vi "Set Protocol Data.vi"(7 "Operation":T1, 8 "error in (no error)":errorcluster, 10 "Protocols.lvlib:Protocol Parent.lvclass":refnum<class "Protocol Parent.lvclass">, 11 "Listener In.lvclass":refnum<class "Listener.lvclass"> caption="Listener") -> (0 "error out":errorcluster, 3 "Listener Out.lvclass":refnum<class "Listener.lvclass">)   [LabVIEW 2023, in "Listener.lvclass"]
uses:
  Listener.lvclass
  TCP/TCP.lvclass
  UDP/UDP.lvclass
  ListenerClassControls/TCP Data Structure.ctl
  ListenerClassControls/UDP Data Structure.ctl
  AK TCP/AK TCP.lvclass
  ListenerClassControls/AK TCP Data Structure.ctl
  ListenerClassControls/Protocol.ctl
  Constants.vi
  AK RS-xxx/AK RS-xxx.lvclass
  ListenerClassControls/RS-xxx Data Structure.ctl
  Protocol Parent/Protocol Parent.lvclass
  <vilib>/Instr/_visa.llb/VISA Configure Serial Port (Instr).vi
  ListenerClassControls/Operation.ctl
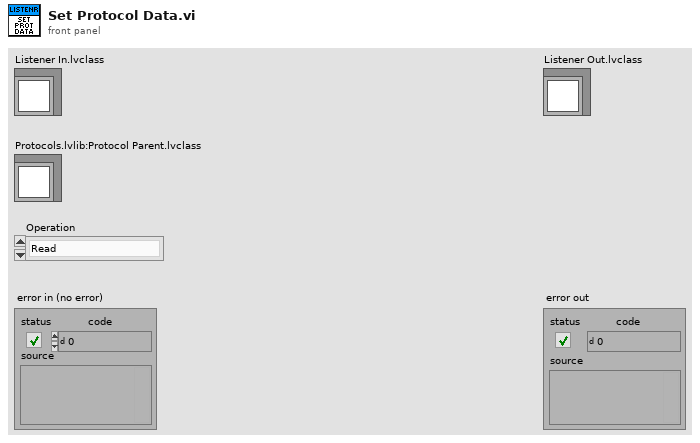
[diagram p1: front panel]
types:
  T1 = typedef "Listener.lvclass/Operation.ctl" = enum16{"Read", "Write"}
  T2 = typedef "Listener.lvclass/Protocol.ctl" = enum16{"RS-XXX", "AK RS-XXX", "VISA", "TCPIP", "AK TCPIP", "UDP", "GPIB ConvBox"}
  T3 = typedef "Listener.lvclass/AK TCP Data Structure.ctl" = cluster{"TCP|IP connection ID":refnum<k5>, "IP Address":string, "Port":u16, "Data":string, "Current Command Code":string}
  T4 = typedef "Listener.lvclass/TCP Data Structure.ctl" = cluster{"TCP|IP connection ID":refnum<k5>, "IP Address":string, "Port":u16, "Data":string}
  T5 = typedef "Listener.lvclass/UDP Data Structure.ctl" = cluster{"UDP connection ID":refnum<k16>, "Local Address":string, "Local Port":u16, "Target IP Address":string, "Target Port":u16, "Data":string}
  T6 = typedef "Listener.lvclass/RS-xxx Data Structure.ctl" = cluster{"Virtual COM Port Settings 1":cluster{"Port":string, "Baud Rate":u32, "Data Bits":u16, "Parity":enum16{"None", "Odd", "Even", "Mark", "Space"}, "Stop Bits":u16, "Flow Control":u16, "XON":enum16{"NUL", "SOH", "STX", "ETX", "EOT", "ENQ", "ACK", "BEL", "BS", "HT", "LF", "VT", "FF", "CR", "SO", "SI", "DLE", "DC1", "DC2", "DC3", "DC4", "NAK", "SYN", "ETB", "CAN", "EM", "SUB", "ESC", "FS", "GS", "RS", "US", "SP", "!", "\"", "#", "$", "%", "&", "'", "(", ")", "*", "+", ",", "- (-)", ".", "/", "0", "1", "2", "3", "4", "5", "6", "7", "8", "9", ":", ";", "<", "=", ">", "?", "@", "A", "B", "C", "D", "E", "F", "G", "H", "I", "J", "K", "L", "M", "N", "O", "P", "Q", "R", "S", "T", "U", "V", "W", "X", "Y", "Z", "[", "\\", "]", "^", "_", "`", "a", "b", "c", "d", "e", "f", "g", "h", "i", "j", "k", "l", "m", "n", "o", "p", "q", "r", "s", "t", "u", "v", "w", "x", "y", "z", "{", "|", "}", "~"}, "XOFF":enum16{"NUL", "SOH", "STX", "ETX", "EOT", "ENQ", "ACK", "BEL", "BS", "HT", "LF", "VT", "FF", "CR", "SO", "SI", "DLE", "DC1", "DC2", "DC3", "DC4", "NAK", "SYN", "ETB", "CAN", "EM", "SUB", "ESC", "FS", "GS", "RS", "US", "SP", "!", "\"", "#", "$", "%", "&", "'", "(", ")", "*", "+", ",", "- (-)", ".", "/", "0", "1", "2", "3", "4", "5", "6", "7", "8", "9", ":", ";", "<", "=", ">", "?", "@", "A", "B", "C", "D", "E", "F", "G", "H", "I", "J", "K", "L", "M", "N", "O", "P", "Q", "R", "S", "T", "U", "V", "W", "X", "Y", "Z", "[", "\\", "]", "^", "_", "`", "a", "b", "c", "d", "e", "f", "g", "h", "i", "j", "k", "l", "m", "n", "o", "p", "q", "r", "s", "t", "u", "v", "w", "x", "y", "z", "{", "|", "}", "~"}, "End Read on Termination Character":bool, "End Write on Termination Character":bool, "Termination Character":u8}, "Virtual COM Port Settings 2":cluster{"Port":string, "Baud Rate":u32, "Data Bits":u16, "Parity":enum16{"None", "Odd", "Even", "Mark", "Space"}, "Stop Bits":u16, "Flow Control":u16, "XON":enum16{"NUL", "SOH", "STX", "ETX", "EOT", "ENQ", "ACK", "BEL", "BS", "HT", "LF", "VT", "FF", "CR", "SO", "SI", "DLE", "DC1", "DC2", "DC3", "DC4", "NAK", "SYN", "ETB", "CAN", "EM", "SUB", "ESC", "FS", "GS", "RS", "US", "SP", "!", "\"", "#", "$", "%", "&", "'", "(", ")", "*", "+", ",", "- (-)", ".", "/", "0", "1", "2", "3", "4", "5", "6", "7", "8", "9", ":", ";", "<", "=", ">", "?", "@", "A", "B", "C", "D", "E", "F", "G", "H", "I", "J", "K", "L", "M", "N", "O", "P", "Q", "R", "S", "T", "U", "V", "W", "X", "Y", "Z", "[", "\\", "]", "^", "_", "`", "a", "b", "c", "d", "e", "f", "g", "h", "i", "j", "k", "l", "m", "n", "o", "p", "q", "r", "s", "t", "u", "v", "w", "x", "y", "z", "{", "|", "}", "~"}, "XOFF":enum16{"NUL", "SOH", "STX", "ETX", "EOT", "ENQ", "ACK", "BEL", "BS", "HT", "LF", "VT", "FF", "CR", "SO", "SI", "DLE", "DC1", "DC2", "DC3", "DC4", "NAK", "SYN", "ETB", "CAN", "EM", "SUB", "ESC", "FS", "GS", "RS", "US", "SP", "!", "\"", "#", "$", "%", "&", "'", "(", ")", "*", "+", ",", "- (-)", ".", "/", "0", "1", "2", "3", "4", "5", "6", "7", "8", "9", ":", ";", "<", "=", ">", "?", "@", "A", "B", "C", "D", "E", "F", "G", "H", "I", "J", "K", "L", "M", "N", "O", "P", "Q", "R", "S", "T", "U", "V", "W", "X", "Y", "Z", "[", "\\", "]", "^", "_", "`", "a", "b", "c", "d", "e", "f", "g", "h", "i", "j", "k", "l", "m", "n", "o", "p", "q", "r", "s", "t", "u", "v", "w", "x", "y", "z", "{", "|", "}", "~"}, "End Read on Termination Character":bool, "End Write on Termination Character":bool, "Termination Character":u8}, "Data":string, "Data Length":u32}
  T7 = typedef "Protocols.lvlib/Protocol Parent.lvclass/Base Protocol Type.ctl" = enum16{"RS-XXX", "VISA", "TCPIP", "UDP", "GPIB ConvBox"}
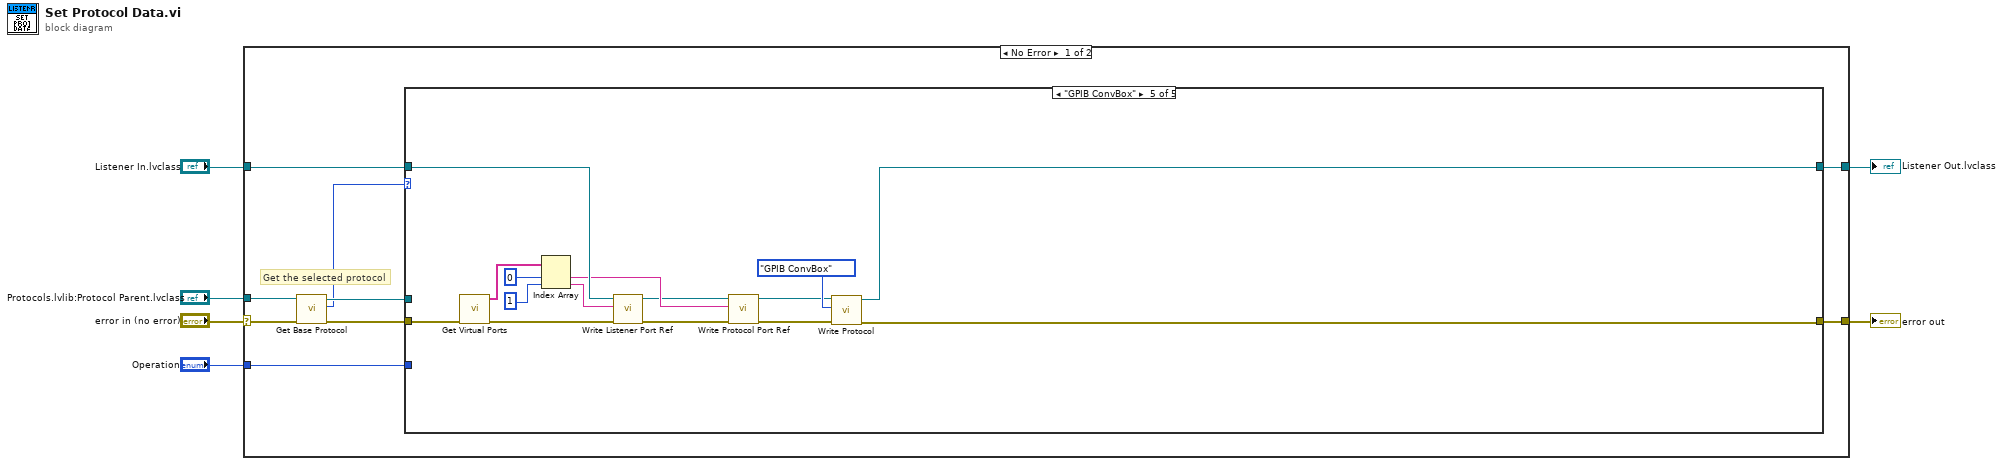
[diagram p0: block diagram]
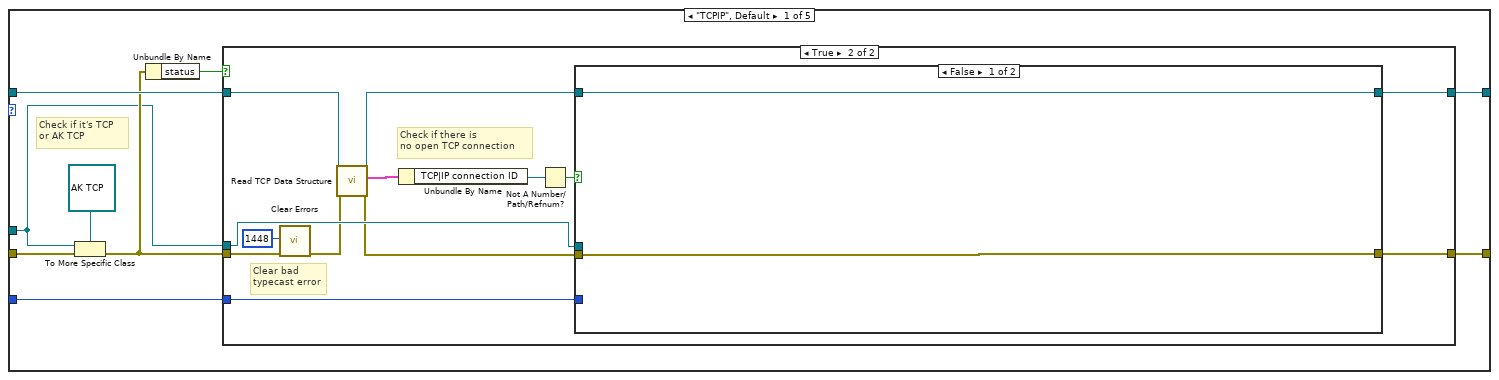
[diagram p2: hidden frame]
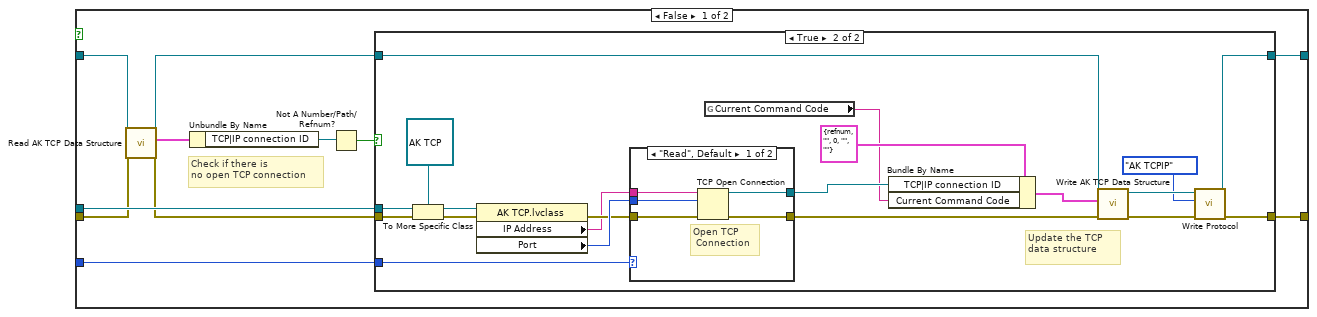
[diagram p3: hidden frame]
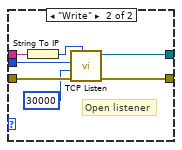
[diagram p5: hidden frame]
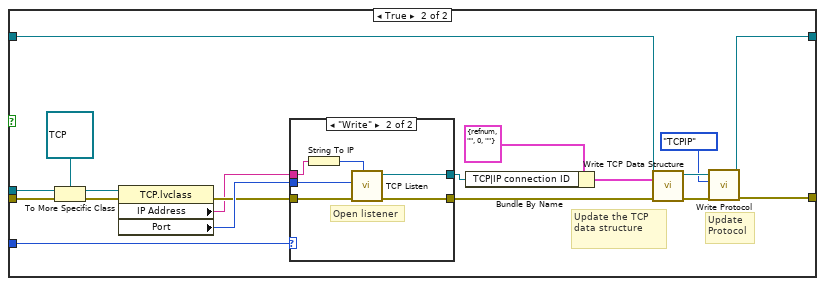
[diagram p6: hidden frame]
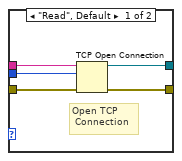
[diagram p7: hidden frame]
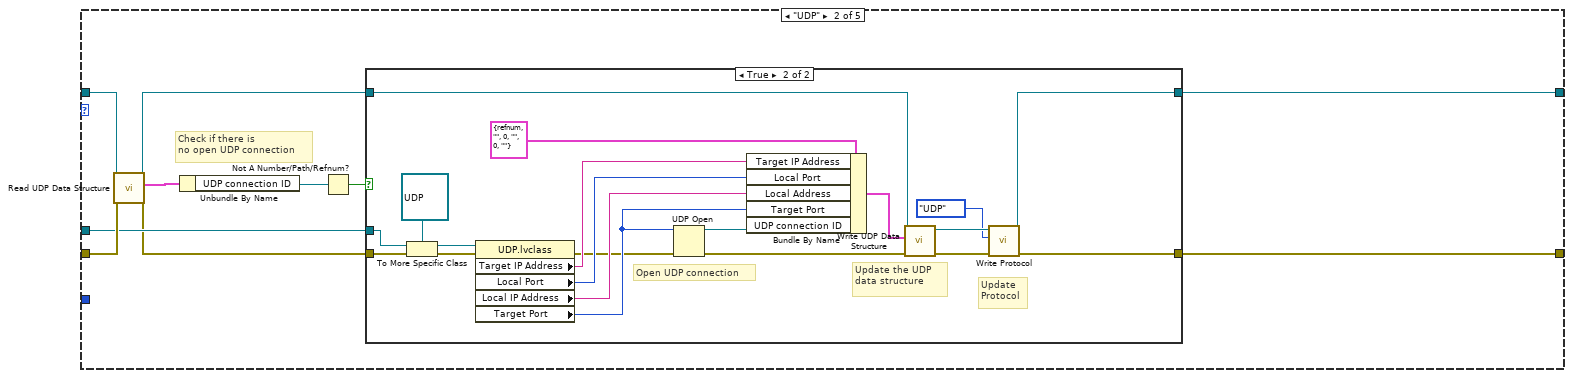
[diagram p8: hidden frame]
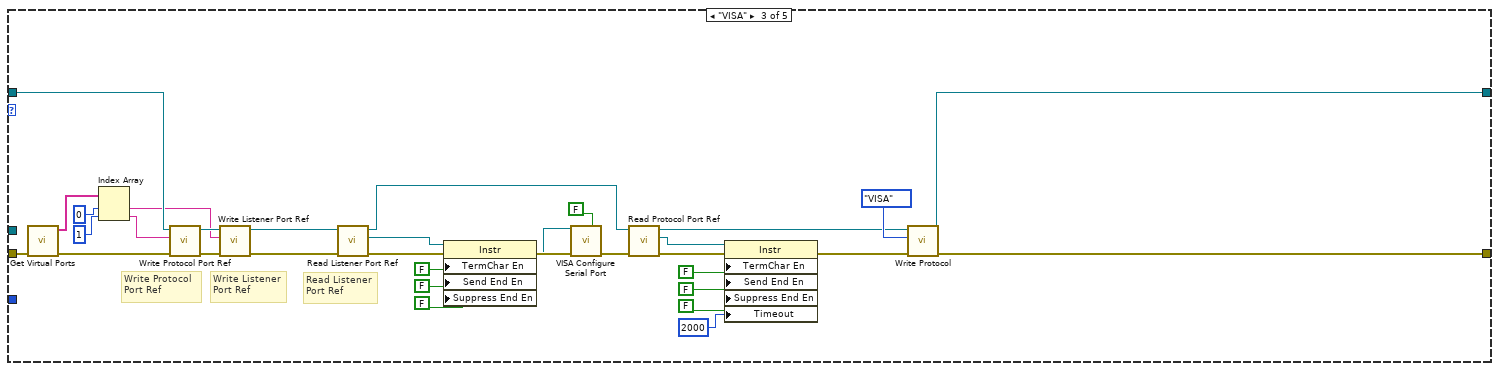
[diagram p10: hidden frame]
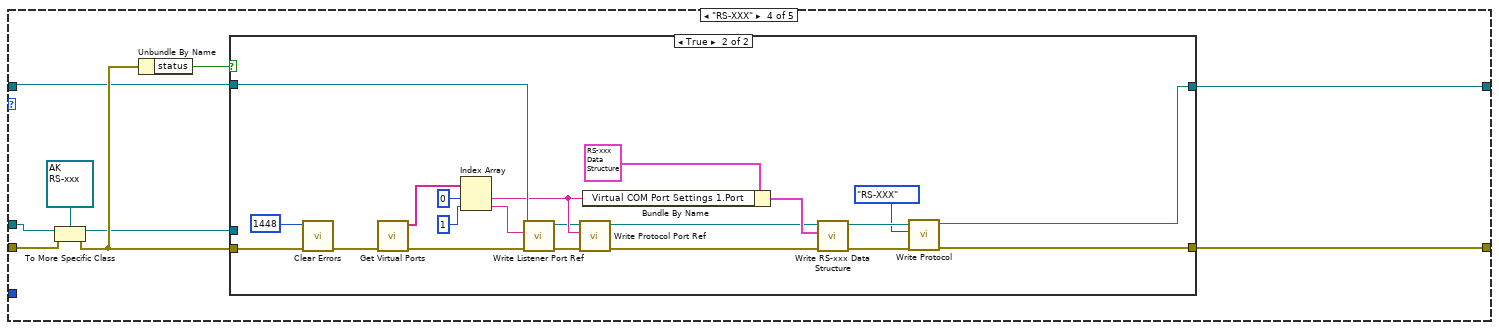
[diagram p11: hidden frame]
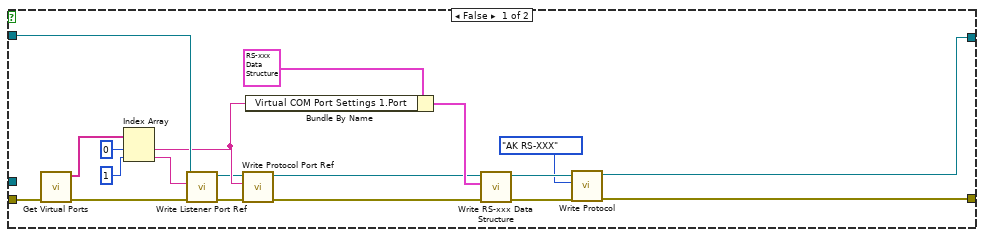
[diagram p12: hidden frame]
diagram:
  n1 = case shown="No Error" "error in (no error)" {
    selector: "error in (no error)" -> [w13 w245]
    tunnel: [w12 w245] -> w5
    tunnel: "Protocols.lvlib:Protocol Parent.lvclass" -> [w14 _]
    tunnel: "Listener In.lvclass" -> [w7 w244]
    tunnel: [w9 w244] -> w2
    tunnel: "Operation" -> [w8 _]
    frame No Error {
      # "Get the selected protocol"
      n2 = call-dynamic "Get Base Protocol.vi"("error in (no error)"=w13, "Protocol Parent in"=w14) -> ("error out"=w11:errorcluster, "Protocol out"=w10:T7, "Protocol Parent out"=w15:refnum<class "Protocol Parent.lvclass">)  [unwired: 7 in]
      n3 = case shown="\"GPIB ConvBox\"" w10 {
        tunnel: w15 -> [w16 w118 _ w181 _]
        tunnel: w11 -> [w20 w120 w179 w188 w243]
        tunnel: [w23 w123 w165 w183 w242] -> w12
        tunnel: w7 -> [w22 w119 w154 w184 w236]
        tunnel: [w24 w124 w178 w182 w241] -> w9
        tunnel: w8 -> [w21 _ _ _ _]
        frame "TCPIP", Default {
          # "Check if it's TCP \nor AK TCP"
          n4 = To More Specific Class(target class=refnum<class "AK TCP.lvclass"> refnum ("Protocols.lvlib:AK TCP.lvclass"), reference=w16, error in=w20) -> (error out=w19:errorcluster)  [unwired: 1 out]
          n5 = Unbundle By Name(w19) -> ("status"=w18:bool)
          n6 = case shown="True" w18 {
            tunnel: w16 -> [w35 w82]
            tunnel: [w34 w81] -> w24
            tunnel: [w33 w80] -> w23
            tunnel: w22 -> [w30 w78]
            tunnel: w19 -> [w28 w77]
            tunnel: w21 -> [w31 w72]
            frame False {
              # "Check if there is \nno open TCP connection"
              n7 = call-dynamic "Read AK TCP Data Structure.vi"("error in (no error)"=w28, "Listener in"=w30) -> ("error out"=w27:errorcluster, "TCP|IP Data Structure"=w26:T3, "Listener out"=w29:refnum<class "Listener.lvclass">)  [unwired: 7 in]
              n8 = Unbundle By Name(w26) -> ("TCP|IP connection ID"=w25:refnum<k5>)
              n9 = Not A Number/Path/Refnum?(number/path/refnum=w25) -> (NaN/Path/Refnum?=w32:bool)
              n10 = case shown="True" w32 {
                tunnel: w35 -> [_ w57]
                tunnel: [w37 w38] -> w34
                tunnel: [w36 w41] -> w33
                tunnel: w27 -> [w36 w54]
                tunnel: w29 -> [w37 w43]
                tunnel: w31 -> [_ w53]
                frame False {
                }
                frame True {
                  # "Update the TCP \ndata structure"
                  n11 = To More Specific Class(target class=refnum<class "AK TCP.lvclass"> refnum ("Protocols.lvlib:AK TCP.lvclass"), reference=w57, error in=w54) -> (specific class reference=w56:refnum<class "AK TCP.lvclass">, error out=w55:errorcluster)
                  n12 = property class="AK TCP.lvclass"(reference=w56, error in=w55) -> (error out=w51:errorcluster, "IP Address"=w50:string, "Port"=w52:u16)  [unwired: 1 out]
                  n13 = case shown="\"Read\", Default" w53 {
                    tunnel: w52 -> [w62 w64]
                    tunnel: w51 -> [w61 w69]
                    tunnel: w50 -> [w60 w68]
                    tunnel: [w59 w65] -> w45
                    tunnel: [w58 w66] -> w49
                    frame "Read", Default {
                      # "Open TCP\n Connection"
                      n14 = TCP Open Connection(address=w60, remote port or service name=w62, error in (no error)=w61) -> (connection ID=w58:refnum<k5>, error out=w59:errorcluster)  [unwired: 2 in]
                    }
                    frame "Write" {
                      # "Open listener"
                      n15 = String To IP(1:w68) -> (0:w67:u32)
                      n16 = call <vilib>:"TCP Listen.vi"("net address"=w67, "error in (no error)"=w69, "timeout ms (wait forever: -1)"=30000, "port"=w64) -> ("error out"=w65:errorcluster, "connection ID"=w66:refnum<k5>)  [unwired: 3 in, 3 out]
                    }
                  }
                  n17 = global read "Constants.vi" "Current Command Code"() -> (w46:string)
                  n18 = Bundle By Name(cluster=T3 {"TCP|IP connection ID"=refnum, "IP Address"="", "Port"=0, "Data"="", "Current Command Code"=""} ("TCP|IP Data Structure"), "TCP|IP connection ID"=w49, "Current Command Code"=w46) -> (w44:T3)
                  n19 = call-dynamic "Write AK TCP Data Structure.vi"("error in (no error)"=w45, "TCP|IP Data Structure"=w44, "Listener in"=w43) -> ("error out"=w42:errorcluster, "Listener out"=w40:refnum<class "Listener.lvclass">)  [unwired: 7 in]
                  n20 = call-dynamic "Write Protocol.vi"("error in (no error)"=w42, "Protocol"=Protocol."AK TCPIP", "Listener in"=w40) -> ("error out"=w41:errorcluster, "Listener out"=w38:refnum<class "Listener.lvclass">)  [unwired: 7 in]
                }
              }
            }
            frame True {
              # "Clear bad \ntypecast error"
              # "Check if there is \nno open TCP connection"
              n21 = call <vilib>:"Clear Errors.vi"("error in (no error)"=w77, "specific error code to clear (0: all)"=1448) -> ("error out"=w71:errorcluster)  [unwired: 4 in, 1 out]
              n22 = call-dynamic "Read TCP Data Structure.vi"("error in (no error)"=w71, "Listener in"=w78) -> ("error out"=w76:errorcluster, "TCP|IP Data Structure"=w75:T4, "Listener out"=w74:refnum<class "Listener.lvclass">)  [unwired: 7 in]
              n23 = Unbundle By Name(w75) -> ("TCP|IP connection ID"=w79:refnum<k5>)
              n24 = Not A Number/Path/Refnum?(number/path/refnum=w79) -> (NaN/Path/Refnum?=w73:bool)
              n25 = case shown="False" w73 {
                tunnel: w82 -> [_ w102]
                tunnel: [w84 w86] -> w81
                tunnel: [w83 w87] -> w80
                tunnel: w76 -> [w83 w98]
                tunnel: w74 -> [w84 w91]
                tunnel: w72 -> [_ w97]
                frame False {
                }
                frame True {
                  # "Update \nProtocol"
                  # "Update the TCP \ndata structure"
                  n26 = To More Specific Class(target class=refnum<class "TCP.lvclass"> refnum ("Protocols.lvlib:TCP.lvclass"), reference=w102, error in=w98) -> (specific class reference=w101:refnum<class "TCP.lvclass">, error out=w100:errorcluster)
                  n27 = property class="TCP.lvclass"(reference=w101, error in=w100) -> (error out=w95:errorcluster, "IP Address"=w94:string, "Port"=w96:u16)  [unwired: 1 out]
                  n28 = case shown="\"Write\"" w97 {
                    tunnel: w96 -> [w108 w113]
                    tunnel: w95 -> [w107 w114]
                    tunnel: w94 -> [w106 w112]
                    tunnel: [w105 w109] -> w92
                    tunnel: [w104 w110] -> w93
                    frame "Read", Default {
                      # "Open TCP\n Connection"
                      n29 = TCP Open Connection(address=w106, remote port or service name=w108, error in (no error)=w107) -> (connection ID=w104:refnum<k5>, error out=w105:errorcluster)  [unwired: 2 in]
                    }
                    frame "Write" {
                      # "Open listener"
                      n30 = String To IP(1:w112) -> (0:w111:u32)
                      n31 = call <vilib>:"TCP Listen.vi"("net address"=w111, "error in (no error)"=w114, "port"=w113) -> ("error out"=w109:errorcluster, "connection ID"=w110:refnum<k5>)  [unwired: 4 in, 3 out]
                    }
                  }
                  n32 = Bundle By Name(cluster=T4 {"TCP|IP connection ID"=refnum, "IP Address"="", "Port"=0, "Data"=""} ("TCP|IP Data Structure"), "TCP|IP connection ID"=w93) -> (w90:T4)
                  n33 = call-dynamic "Write TCP Data Structure.vi"("error in (no error)"=w92, "TCP|IP Data Structure"=w90, "Listener in"=w91) -> ("error out"=w89:errorcluster, "Listener out"=w88:refnum<class "Listener.lvclass">)  [unwired: 7 in]
                  n34 = call-dynamic "Write Protocol.vi"("error in (no error)"=w89, "Protocol"=Protocol."TCPIP", "Listener in"=w88) -> ("error out"=w87:errorcluster, "Listener out"=w86:refnum<class "Listener.lvclass">)  [unwired: 7 in]
                }
              }
            }
          }
        }
        frame "UDP" {
          # "Check if there is \nno open UDP connection"
          n35 = call-dynamic "Read UDP Data Structure.vi"("error in (no error)"=w120, "Listener in"=w119) -> ("error out"=w116:errorcluster, "UDP Data Structure"=w117:T5, "Listener out"=w115:refnum<class "Listener.lvclass">)  [unwired: 7 in]
          n36 = Unbundle By Name(w117) -> ("UDP connection ID"=w121:refnum<k16>)
          n37 = Not A Number/Path/Refnum?(number/path/refnum=w121) -> (NaN/Path/Refnum?=w122:bool)
          n38 = case shown="True" w122 {
            tunnel: w116 -> [w126 w146]
            tunnel: w118 -> [_ w144]
            tunnel: w115 -> [w125 w133]
            tunnel: [w125 w127] -> w124
            tunnel: [w126 w128] -> w123
            frame False {
            }
            frame True {
              # "Update \nProtocol"
              # "Update the UDP \ndata structure"
              # "Open UDP connection"
              n39 = To More Specific Class(target class=refnum<class "UDP.lvclass"> refnum ("Protocols.lvlib:UDP.lvclass"), reference=w144, error in=w146) -> (specific class reference=w138:refnum<class "UDP.lvclass">, error out=w143:errorcluster)
              n40 = property class="UDP.lvclass"(reference=w138, error in=w143) -> (error out=w136:errorcluster, "Target IP Address"=w142:string, "Local Port"=w141:u16, "Local IP Address"=w140:string, "Target Port"=w137:u16)  [unwired: 1 out]
              n41 = UDP Open(8:w136, 11:w137) -> (port=w135:refnum<k16>, 0:w134:errorcluster)  [unwired: 3 in, 1 out]
              n42 = Bundle By Name(cluster=T5 {"UDP connection ID"=refnum, "Local Address"="", "Local Port"=0, "Target IP Address"="", "Target Port"=0, "Data"=""} ("UDP Data Structure"), "Target IP Address"=w142, "Local Port"=w141, "Local Address"=w140, "Target Port"=w137, "UDP connection ID"=w135) -> (w132:T5)
              n43 = call-dynamic "Write UDP Data Structure.vi"("error in (no error)"=w134, "UDP Data Structure"=w132, "Listener in"=w133) -> ("error out"=w131:errorcluster, "Listener out"=w130:refnum<class "Listener.lvclass">)  [unwired: 7 in]
              n44 = call-dynamic "Write Protocol.vi"("error in (no error)"=w131, "Protocol"=Protocol."UDP", "Listener in"=w130) -> ("error out"=w128:errorcluster, "Listener out"=w127:refnum<class "Listener.lvclass">)  [unwired: 7 in]
            }
          }
        }
        frame "VISA" {
          # "Read Listener\nPort Ref"
          # "Write Listener\nPort Ref"
          # "Write Protocol\nPort Ref"
          n45 = call "Get Virtual Ports.vi"("error in (no error)"=w179) -> ("error out"=w155:errorcluster, "Serial Ports out"=w174:string[])  [unwired: 9 in]
          n46 = Index Array(array=w174, index #1=0 ("index"), index #2=1 ("index")) -> (element #1=w152:string, element #2=w153:string)
          n47 = call "Write Protocol Port Ref.vi"("error in (no error)"=w155, "Protocol Port Ref"=w153, "Listener in"=w154) -> ("error out"=w157:errorcluster, "Listener out"=w156:refnum<class "Listener.lvclass">)  [unwired: 7 in]
          n48 = call "Write Listener Port Ref.vi"("error in (no error)"=w157, "Listener Port Ref"=w152, "Listener in"=w156) -> ("error out"=w160:errorcluster, "Listener out"=w161:refnum<class "Listener.lvclass">)  [unwired: 7 in]
          n49 = call "Read Listener Port Ref.vi"("error in (no error)"=w160, "Listener in"=w161) -> ("error out"=w159:errorcluster, "Listener Port Ref"=w158:refnum<visa-resource-name>, "Listener out"=w150:refnum<class "Listener.lvclass">)  [unwired: 7 in]
          n50 = property class="Instr"(reference=w158, error in=w159, "TermChar En"=FALSE ("Message Based Settings:Termination Character Enable"), "Send End En"=FALSE ("Message Based Settings:Send End Enable"), "Suppress End En"=FALSE ("Message Based Settings:Suppress End Enable")) -> (reference out=w163:refnum<visa-resource-name>, error out=w164:errorcluster)
          n51 = call-poly "VISA Configure Serial Port"("VISA resource name"=w163, "Enable Termination\nChar (T)"=FALSE ("Enable Termination\nChar (T)"), "error in (no error)"=w164) -> ("error out"=w151:errorcluster)  [unwired: 11 in, 1 out]
          n52 = call "Read Protocol Port Ref.vi"("error in (no error)"=w151, "Listener in"=w150) -> ("error out"=w148:errorcluster, "Protocol Port Ref"=w149:refnum<visa-resource-name>, "Listener out"=w147:refnum<class "Listener.lvclass">)  [unwired: 7 in]
          n53 = property class="Instr"(reference=w149, error in=w148, "TermChar En"=FALSE ("Message Based Settings:Termination Character Enable"), "Send End En"=FALSE ("Message Based Settings:Send End Enable"), "Suppress End En"=FALSE ("Message Based Settings:Suppress End Enable"), "Timeout"=u32 2000 ("General Settings:Timeout Value")) -> (error out=w162:errorcluster)  [unwired: 1 out]
          n54 = call-dynamic "Write Protocol.vi"("error in (no error)"=w162, "Protocol"=Protocol."VISA", "Listener in"=w147) -> ("error out"=w165:errorcluster, "Listener out"=w178:refnum<class "Listener.lvclass">)  [unwired: 7 in]
        }
        frame "RS-XXX" {
          n55 = To More Specific Class(target class=refnum<class "AK RS-xxx.lvclass"> refnum ("Protocols.lvlib:AK RS-xxx.lvclass"), reference=w181, error in=w188) -> (specific class reference=w180:refnum<class "AK RS-xxx.lvclass">, error out=w185:errorcluster)
          n56 = Unbundle By Name(w185) -> ("status"=w186:bool)
          n57 = case shown="True" w186 {
            tunnel: w185 -> [w207 w210]
            tunnel: w184 -> [w194 w216]
            tunnel: [w205 w227] -> w183
            tunnel: [w203 w225] -> w182
            tunnel: w180 -> [_ _]
            frame False {
              n58 = call "Get Virtual Ports.vi"("error in (no error)"=w207) -> ("error out"=w196:errorcluster, "Serial Ports out"=w198:string[])  [unwired: 9 in]
              n59 = Index Array(array=w198, index #1=0 ("index"), index #2=1 ("index")) -> (element #1=w192:string, element #2=w195:string)
              n60 = call "Write Listener Port Ref.vi"("error in (no error)"=w196, "Listener Port Ref"=w195, "Listener in"=w194) -> ("error out"=w193:errorcluster, "Listener out"=w191:refnum<class "Listener.lvclass">)  [unwired: 7 in]
              n61 = call "Write Protocol Port Ref.vi"("error in (no error)"=w193, "Protocol Port Ref"=w192, "Listener in"=w191) -> ("error out"=w190:errorcluster, "Listener out"=w189:refnum<class "Listener.lvclass">)  [unwired: 7 in]
              n62 = Bundle By Name(cluster=T6 {"Virtual COM Port Settings 1"={"Port"="COM1", "Baud Rate"=9600, "Data Bits"=8, "Parity"=enum."None", "Stop Bits"=10, "Flow Control"=0, "XON"=enum."DC1", "XOFF"=enum."DC3", "End Read on Termination Character"=FALSE, "End Write on Termination Character"=FALSE, "Termination Character"=10}, "Virtual COM Port Settings 2"={"Port"="COM1", "Baud Rate"=9600, "Data Bits"=8, "Parity"=enum."None", "Stop Bits"=10, "Flow Control"=0, "XON"=enum."DC1", "XOFF"=enum."DC3", "End Read on Termination Character"=FALSE, "End Write on Termination Character"=FALSE, "Termination Character"=10}, "Data"="", "Data Length"=0} ("RS-xxx Data Structure"), "Virtual COM Port Settings 1.Port"=w192) -> (w197:T6)
              n63 = call-dynamic "Write RS-xxx Data Structure.vi"("error in (no error)"=w190, "RS-xxx Data Structure"=w197, "Listener in"=w189) -> ("error out"=w206:errorcluster, "Listener out"=w204:refnum<class "Listener.lvclass">)  [unwired: 7 in]
              n64 = call-dynamic "Write Protocol.vi"("error in (no error)"=w206, "Protocol"=Protocol."AK RS-XXX", "Listener in"=w204) -> ("error out"=w205:errorcluster, "Listener out"=w203:refnum<class "Listener.lvclass">)  [unwired: 7 in]
            }
            frame True {
              n65 = call <vilib>:"Clear Errors.vi"("error in (no error)"=w210, "specific error code to clear (0: all)"=1448) -> ("error out"=w209:errorcluster)  [unwired: 4 in, 1 out]
              n66 = call "Get Virtual Ports.vi"("error in (no error)"=w209) -> ("error out"=w218:errorcluster, "Serial Ports out"=w220:string[])  [unwired: 9 in]
              n67 = Index Array(array=w220, index #1=0 ("index"), index #2=1 ("index")) -> (element #1=w214:string, element #2=w217:string)
              n68 = call "Write Listener Port Ref.vi"("error in (no error)"=w218, "Listener Port Ref"=w217, "Listener in"=w216) -> ("error out"=w215:errorcluster, "Listener out"=w213:refnum<class "Listener.lvclass">)  [unwired: 7 in]
              n69 = call "Write Protocol Port Ref.vi"("error in (no error)"=w215, "Protocol Port Ref"=w214, "Listener in"=w213) -> ("error out"=w212:errorcluster, "Listener out"=w211:refnum<class "Listener.lvclass">)  [unwired: 7 in]
              n70 = Bundle By Name(cluster=T6 {"Virtual COM Port Settings 1"={"Port"="COM1", "Baud Rate"=9600, "Data Bits"=8, "Parity"=enum."None", "Stop Bits"=10, "Flow Control"=0, "XON"=enum."DC1", "XOFF"=enum."DC3", "End Read on Termination Character"=FALSE, "End Write on Termination Character"=FALSE, "Termination Character"=10}, "Virtual COM Port Settings 2"={"Port"="COM1", "Baud Rate"=9600, "Data Bits"=8, "Parity"=enum."None", "Stop Bits"=10, "Flow Control"=0, "XON"=enum."DC1", "XOFF"=enum."DC3", "End Read on Termination Character"=FALSE, "End Write on Termination Character"=FALSE, "Termination Character"=10}, "Data"="", "Data Length"=0} ("RS-xxx Data Structure"), "Virtual COM Port Settings 1.Port"=w214) -> (w219:T6)
              n71 = call-dynamic "Write RS-xxx Data Structure.vi"("error in (no error)"=w212, "RS-xxx Data Structure"=w219, "Listener in"=w211) -> ("error out"=w228:errorcluster, "Listener out"=w226:refnum<class "Listener.lvclass">)  [unwired: 7 in]
              n72 = call-dynamic "Write Protocol.vi"("error in (no error)"=w228, "Protocol"=Protocol."RS-XXX", "Listener in"=w226) -> ("error out"=w227:errorcluster, "Listener out"=w225:refnum<class "Listener.lvclass">)  [unwired: 7 in]
            }
          }
        }
        frame "GPIB ConvBox" {
          n73 = call "Get Virtual Ports.vi"("error in (no error)"=w243) -> ("error out"=w234:errorcluster, "Serial Ports out"=w237:string[])  [unwired: 9 in]
          n74 = Index Array(array=w237, index #1=0 ("index"), index #2=1 ("index")) -> (element #1=w233:string, element #2=w235:string)
          n75 = call "Write Listener Port Ref.vi"("error in (no error)"=w234, "Listener Port Ref"=w235, "Listener in"=w236) -> ("error out"=w232:errorcluster, "Listener out"=w231:refnum<class "Listener.lvclass">)  [unwired: 7 in]
          n76 = call "Write Protocol Port Ref.vi"("error in (no error)"=w232, "Protocol Port Ref"=w233, "Listener in"=w231) -> ("error out"=w229:errorcluster, "Listener out"=w230:refnum<class "Listener.lvclass">)  [unwired: 7 in]
          n77 = call-dynamic "Write Protocol.vi"("error in (no error)"=w229, "Protocol"=Protocol."GPIB ConvBox", "Listener in"=w230) -> ("error out"=w242:errorcluster, "Listener out"=w241:refnum<class "Listener.lvclass">)  [unwired: 7 in]
        }
      }
    }
    frame Error {
    }
  }
  "Listener Out.lvclass" <- w2
  "error out" <- w5
